vi "Teleop.vi"(10 "Match Info":T1={"Autonomous Elapsed Seconds"=0.0, "TeleOp Elapsed Seconds"=0.0, "Disabled Elapsed Seconds"=0.0, "Visited Autonomous"=FALSE, "Visited TeleOp"=FALSE, "Visited Disabled"=FALSE, "Autonomous Settings"={"Autonomous Style"=enum."Independent", "VI Refnum"=refnum}}, 11 "Call Context":T2) -> ()   [LabVIEW 2016]
doc: "This VI is called for each TeleOp packet received from the DS where the robot is not disabled. It is often used to read from the joysticks and update I/O or to update setpoints for timed control loops. It should complete and return within 20 milliseconds or it may miss DS packets."
uses:
  <vilib>/Rock Robotics/WPI/DriverStation/WPI_DriverStationDerivedRobotMode.ctl
  <vilib>/Rock Robotics/WPI/DriverStation/WPI_DriverStationMatch Info.ctl
  <vilib>/Rock Robotics/WPI/ThirdParty/Sensors/Pigeon/CTRE_PigeonIMU_PigeonState.ctl
  <vilib>/Rock Robotics/WPI/Utilities/WPI_GetSetVariantRefNum.vi
  <vilib>/Rock Robotics/Network Tables/NT Write Numeric Array.vi
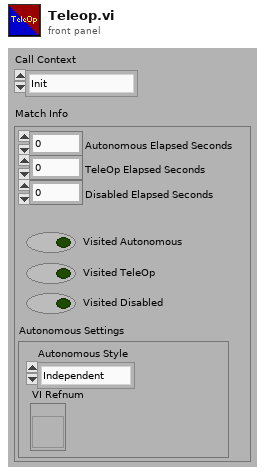
[diagram p1: front panel]
types:
  T1 = typedef "WPI_DriverStationMatch Info.ctl" = cluster{"Autonomous Elapsed Seconds":dbl, "TeleOp Elapsed Seconds":dbl, "Disabled Elapsed Seconds":dbl, "Visited Autonomous":bool, "Visited TeleOp":bool, "Visited Disabled":bool, "Autonomous Settings":cluster{"Autonomous Style":enum16{"Iterative", "Independent"}, "VI Refnum":refnum<vi>}}
  T2 = typedef "WPI_DriverStationDerivedRobotMode.ctl" = enum16{"Init", "Execute", "Stop"}
  T3 = typedef "WPI_RobotDriveDevRef.ctl" = cluster{"DevStatus":errorcluster, "Motors[]":T4[], "Square Inputs":bool, "Max Output":dbl}
  T4 = typedef "WPI_MotorControlDeviceRef.ctl" = cluster{"DeviceStatus":errorcluster, "Type":T5, "PWM":cluster{"PWM Channel":T6, "DeadBand":T7}, "CAN":cluster{"Device Number":u8, "SetOutput VI Ref":variant, "GetOutput VI Ref":variant, "Enable VI Ref":variant, "Disable VI Ref":variant, "Data":variant}, "Invert":bool}
  T5 = typedef "WPI_MotorControlType.ctl" = enum16{"PWM", "CAN"}
  T6 = typedef "FPGA_DIOPWMChannel.ctl" = enum8{"PWM 0", "PWM 1", "PWM 2", "PWM 3", "PWM 4", "PWM 5", "PWM 6", "PWM 7", "PWM 8", "PWM 9", "PWM MXP 0", "PWM MXP 1", "PWM MXP 2", "PWM MXP 3", "PWM MXP 4", "PWM MXP 5", "PWM MXP 6", "PWM MXP 7", "PWM MXP 8", "PWM MXP 9", "Invalid"}
  T7 = typedef "WPI_PWMDeadband.ctl" = cluster{"Name":string, "maxPositivePwm":i32, "minPositivePwm":i32, "centerPwm":i32, "maxNegativePwm":i32, "minNegativePwm":i32, "angularRange":u16}
  T8 = typedef "WPI_JoystickDevRef.ctl" = cluster{"Device":T9}
  T9 = typedef "WPI_JoystickDeviceEnum.ctl" = enum16{"USB 0", "USB 1", "USB 2", "USB 3", "USB 4", "USB 5"}
  T10 = typedef "CTRE_PigeonIMU_DeviceRef.ctl" = cluster{"DeviceStatus":errorcluster, "Device Number":u8, "Type":T11, "Device ID":u32}
  T11 = typedef "CTRE_PigeonIMU_ConnectionType.ctl" = u32
  T12 = typedef "CTRE_PigeonIMU_PigeonState.ctl" = enum16{"NoComm", "Initializing", "Ready", "UserCalibration"}
  T13 = typedef "CTRE_PigeonIMU_GlobalStatus.ctl" = cluster{"PigeonState":T12, "FusedHeading":cluster{"Heading":dbl, "Valid?":bool, "Fusing?":bool}, "YPR":cluster{"Yaw":dbl, "Pitch":dbl, "Roll":dbl}, "Compass":cluster{"Heading":dbl, "Magnitude":dbl, "Absolute Heading":dbl}, "Accelerometer":cluster{"Biased":cluster{"X":i16, "Y":i16, "Z":i16, "Norm":i16}, "Angles":cluster{"XZ Tilt":dbl, "YZ Tilt":dbl, "XY Tilt":dbl}}, "Magnetometer":cluster{"Raw":cluster{"X":i16, "Y":i16, "Z":i16}, "Biased":cluster{"X":i16, "Y":i16, "Z":i16}}, "Gyro":cluster{"X":dbl, "Y":dbl, "Z":dbl, "Norm":dbl}, "6D Quaternian":cluster{"W":dbl, "X":dbl, "Y":dbl, "Z":dbl}, "Temp. (C)":dbl, "UpTime":u32, "StartupStatus":cluster{"ResetCount":i32, "ResetFlags":i32, "FirmwareVersion":i32, "HasReset?":bool}, "Calibration":cluster{"CurrentMode":T14, "LastCalError":i32, "CalBooting?":bool}, "CAN Error":errorcluster, "AccumGyro":cluster{"X":dbl, "Y":dbl, "Z":dbl}}
  T14 = typedef "CTRE_PigeonIMU_CalibrationMode.ctl" = u16
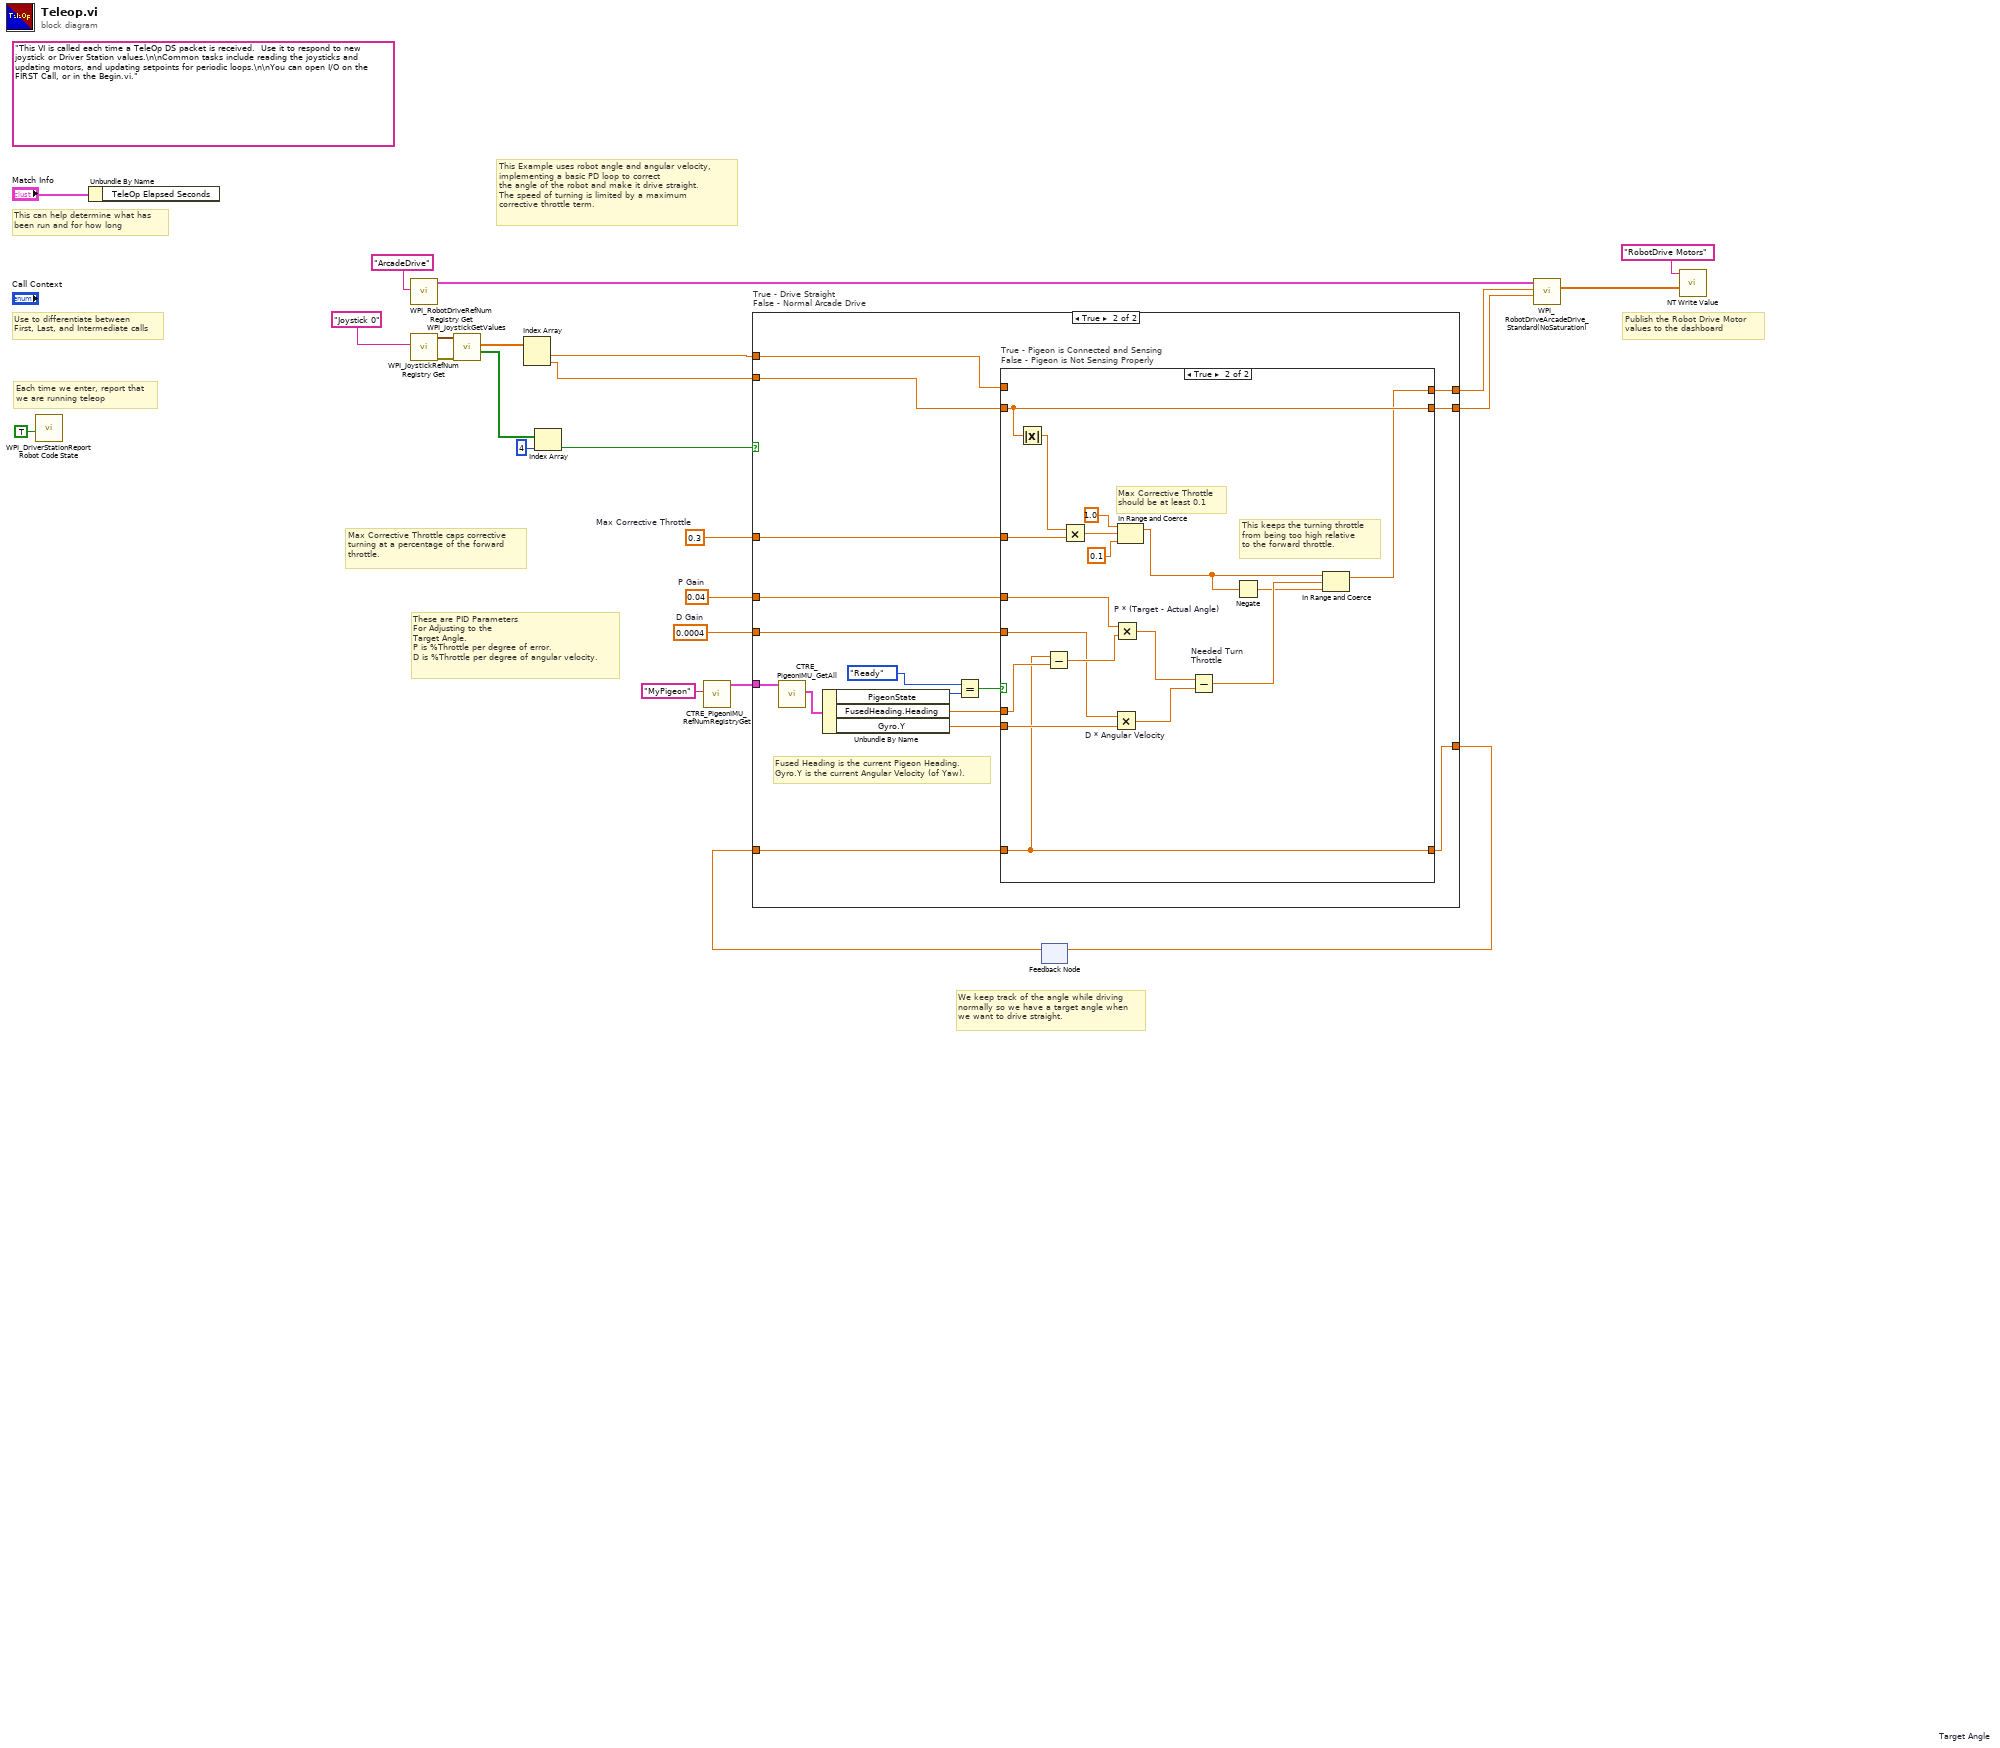
[diagram p0: block diagram]
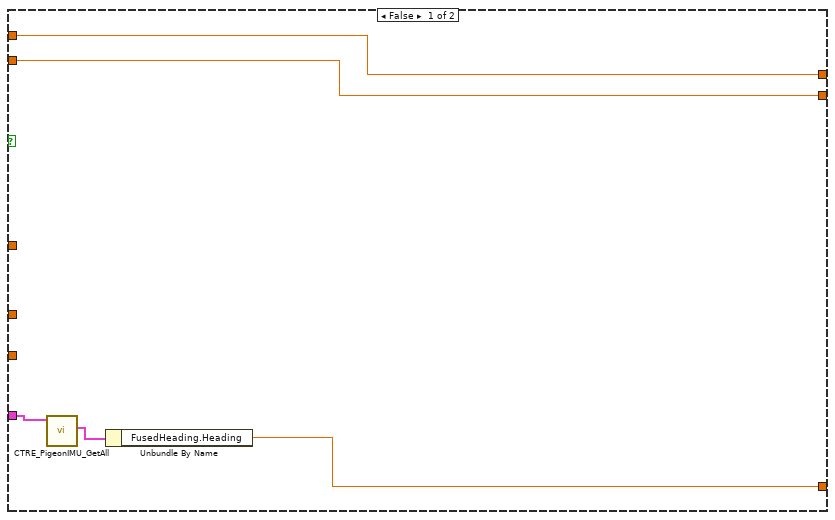
[diagram p2: hidden frame]
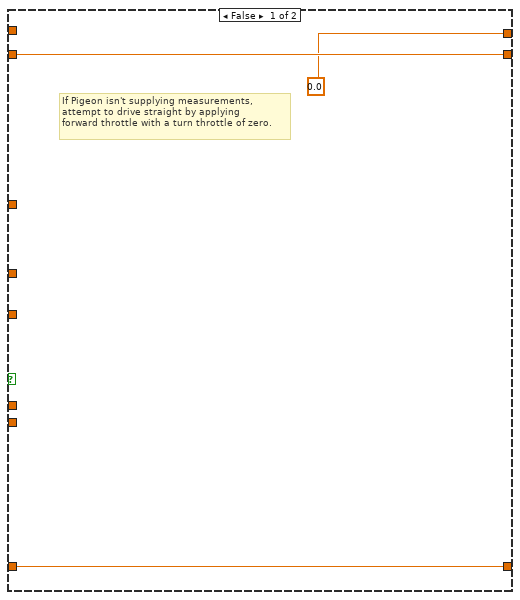
[diagram p3: hidden frame]
diagram:
  w1 = 0.3  # Max Corrective Throttle
  w4 = 0.0004  # D Gain
  w5 = 0.04  # P Gain
  (unwired) "This VI is called each time a TeleOp DS packet is received.  Use it to respond to new joystick or Driver Station values.\n\nCommon tasks include reading the joysticks and updating motors, and updating setpoints for periodic loops.\n\nYou can open I/O on the FIRST Call, or in the Begin.vi."
  # "This Example uses robot angle and angular velocity, \nimplementing a basic PD loop to correct\nthe angle of the robot and make it drive straight.\nThe speed of turning is limited by a maximum \ncorrective throttle term."
  # "Max Corrective Throttle caps corrective\nturning at a percentage of the forward\nthrottle."
  # "We keep track of the angle while driving\nnormally so we have a target angle when\nwe want to drive straight."
  # "These are PID Parameters\nFor Adjusting to the\nTarget Angle.\nP is %Throttle per degree of error.\nD is %Throttle per degree of angular velocity."
  # "Publish the Robot Drive Motor\nvalues to the dashboard"
  # "Each time we enter, report that\nwe are running teleop"
  # "Use to differentiate between\nFirst, Last, and Intermediate calls"
  # "This can help determine what has\nbeen run and for how long"
  n1 = call <vilib>:"WPI_DriverStationReport Robot Code State.vi"("TeleOp"=TRUE ("Autonomous")) -> ()  [unwired: 10 in, 1 out]
  n2 = Unbundle By Name("Match Info") -> ()  [unwired: 1 out]
  n3 = call <vilib>:"WPI_RobotDriveRefNum Registry Get.vi"("refnum name"="ArcadeDrive") -> ("RobotDriveDevRef"=w22:T3)  [unwired: 1 in, 9 out]
  n4 = call <vilib>:"WPI_JoystickRefNum Registry Get.vi"("refnum name"="Joystick 0") -> ("error out"=w7:errorcluster, "JoystickDevRef"=w20:T8)  [unwired: 1 in, 8 out]
  n5 = call <vilib>:"WPI_JoystickGetValues.vi"("error in (no error)"=w7, "JoystickDevRef"=w20) -> ("Buttons"=w11:bool[], "Axes"=w18:dbl[])  [unwired: 5 in, 3 out]
  n6 = Index Array(array=w18) -> (element #1=w15:dbl, element #2=w14:dbl)  [unwired: 2 in]
  n7 = Index Array(array=w11, index=4) -> (element=w9:bool)
  n8 = call "CTRE_PigeonIMU_RefNumRegistryGet.vi"("refnum name"="MyPigeon") -> ("PigeonIMUDevRef"=w6:T10)  [unwired: 9 in, 1 out]
  n9 = feedback #1 "Target Angle"() -> (w2:dbl)  [unwired: 1 in]
  n10 = case "True - Drive Straight\nFalse - Normal Arcade Drive" shown="True" w9 {
    tunnel: w15 -> [w29 w42]
    tunnel: w14 -> [w28 w41]
    tunnel: [w29 w39] -> w12
    tunnel: [w28 w40] -> w13
    tunnel: w6 -> [w27 w44]
    tunnel: w5 -> [_ w33]
    tunnel: w4 -> [_ w32]
    tunnel: [w25 w30] -> w3
    tunnel: w2 -> [_ w35]
    tunnel: w1 -> [_ w31]
    frame False {
      n11 = call "CTRE_PigeonIMU_GetAll.vi"("PigeonIMUDevRef"=w27) -> ("Get All"=w26:T13)  [unwired: 8 in, 2 out]
      n12 = Unbundle By Name(w26) -> ("FusedHeading.Heading"=w25:dbl)
    }
    frame True {
      # "Fused Heading is the current Pigeon Heading.\nGyro.Y is the current Angular Velocity (of Yaw)."
      n13 = call "CTRE_PigeonIMU_GetAll.vi"("PigeonIMUDevRef"=w44) -> ("Get All"=w45:T13)  [unwired: 8 in, 2 out]
      n14 = Unbundle By Name(w45) -> ("PigeonState"=w37:T12, "FusedHeading.Heading"=w36:dbl, "Gyro.Y"=w34:dbl)
      n15 = Equal?(x=CTRE_PigeonIMU_PigeonState."Ready" ("PigeonState"), y=w37) -> (x = y?=w43:bool)
      n16 = case "True - Pigeon is Connected and Sensing\nFalse - Pigeon is Not Sensing Properly" shown="True" w43 {
        tunnel: w42 -> [_ _]
        tunnel: w41 -> [w48 w57]
        tunnel: [w48 w57] -> w40
        tunnel: [0.0 ("upper limit") w50] -> w39
        tunnel: w36 -> [_ w66]
        tunnel: w35 -> [w46 w49]
        tunnel: w34 -> [_ w63]
        tunnel: w33 -> [_ w64]
        tunnel: w32 -> [_ w62]
        tunnel: w31 -> [_ w59]
        tunnel: [w46 w49] -> w30
        frame False {
          # "If Pigeon isn't supplying measurements,\nattempt to drive straight by applying\nforward throttle with a turn throttle of zero."
        }
        frame True {
          # "This keeps the turning throttle\nfrom being too high relative\nto the forward throttle."
          # "Max Corrective Throttle\nshould be at least 0.1"
          n17 = Absolute Value(x=w57) -> (abs(x)=w58:dbl)
          n18 = Subtract(x=w49, y=w66) -> (x-y=w65:dbl)
          n19 = Multiply ("P * (Target - Actual Angle)")(x=w58, y=w59) -> (x*y=w54:dbl)
          n20 = Multiply "D * Angular Velocity"(x=w62, y=w63) -> (x*y=w60:dbl)
          n21 = Multiply "P * (Target - Actual Angle)"(x=w64, y=w65) -> (x*y=w61:dbl)
          n22 = In Range and Coerce(upper limit=1.0, x=w54, lower limit=0.1) -> (coerced(x)=w52:dbl)  [unwired: 1 out]
          n23 = Subtract "Needed Turn \nThrottle"(x=w61, y=w60) -> (x-y=w53:dbl)
          n24 = Negate(x=w52) -> (-x=w51:dbl)
          n25 = In Range and Coerce(upper limit=w52, x=w53, lower limit=w51) -> (coerced(x)=w50:dbl)  [unwired: 1 out]
        }
      }
    }
  }
  n26 = feedback-in #1(w3) -> ()
  n27 = call <vilib>:"WPI_RobotDriveArcadeDrive_Standard(NoSaturation).vi"("Y axis value"=w13, "X axis value"=w12, "RobotDriveDevRef"=w22) -> ("Motor Values"=w17:dbl[])  [unwired: 1 in, 7 out]
  n28 = call-poly <vilib>:"NT Write Value.vi"("Numeric Array"=w17, "Name"="RobotDrive Motors") -> ()  [unwired: 9 in, 1 out]
